vi "Application and database upload.vi"(8 "error in":errorcluster) -> (0 "error out":errorcluster, 1 ".dta file Path 2":path, 2 "Pass?":bool, 3 ".128 file Path 2":path)   [LabVIEW 2009]
uses:
  Digit IO PCI 6503/Digit IO control.ctl
  Global/Global 1.vi
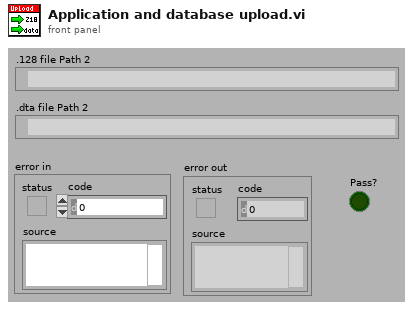
[diagram p1: front panel]
types:
  T1 = typedef "Digit IO control.ctl" = enum16{"Pull X1_4 Low", "Disconnect Pull X1_4 Low", "Down Cylinder", "Disconnect Down Cylinder", "Load X1_1_5", "Disconnect Load X1_1_5", "Measu X1_1_5", "Disconnect Measu X1_1_5", "Measu Z1_1_5", "Disconnect Measu Z1_1_5", "Power X1_1", "Disconnect Power X1_1", "RS232 Power", "Disconnect RS232 Power", "Card Cylinder", "Disconnect Card Cylinder", "Fail LED", "Disconnect Fail LED", "LCA Power", "Disconnect LCA Power", "BeyondCylinderDowndigit", "Disconnect BeyondCylinderDowendigit", "Frequency", "Disconnect Frequency", "Measu Current", "Disconnect Measu Current", "Measu current_1", "Disconnect Measu current_1", "Digit ALL", "Disconnect Digit ALL", "PASS LED", "Disconnect PASS LED", "Load Z1_1_3", "Disconnect Load Z1_1_3", "RS232 Connect", "Disconnect RS232 Connect", "Power Z1_7", "Disconnect Power Z1_7", "Pull Z_1_5  low", "Disconnect Pull Z_1_5  low", "Connect LCA_1", "Disconnect LCA_1", "short LCA", "Disconnect short LCA", "PT100", "Disconnect PT100", "NO connect", "Disconnect NO connect"}
  T2 = enum16{"Initialize", "Uploading 218 file", "Wait APPWAIT", "Uploading dta file", "Wait DBWATI", "Finish"}
  T3 = cluster{".128 file":path, "Appliction firmware file":path, "Data file":path, "Txt path":path, "EXCEL path":path}
  T4 = cluster{"VHEATFUSENOLOADMIN":string, "VHEATFUSELOADMAX":string, "VOVERRIDEDIODEMIN":string, "TDIFFMAX":string, "MEASFREQMAX":string, "MEASFREQMIN":string, "VOVER":string, "VMIDDLE":string, "VUNDER":string, "VNORESET":string, "VRESET":string, "WAITPING":string, "LRFID":string, "RFIDUID":string, "EXTEESIZE":string, "LCUTYPE":string, "LCUSUBTYPE":string, "TEVN":string, "BOOTVER":string, "APPVER":string, "ISLEEPMAX":string, "TSLEEP":string, "APPWAIT":string, "DBWAIT":string}
  T5 = cluster{"People":string, "product  number":string, "Test time":string, "VHeatFuse_noload":string, "VHeatFuse_load":string, "VoverrideDiode":string, "Test firmware upload via X1":string, "TemperAddress":string, "Troom":string, "TLCU":string, "Adjustment factor":string, "MeasuredFreq":string, "I2C communication":string, "Light-emitting diode on Z2":string, "Battery warning/inhibit":string, "Reset by IC10":string, "External EEPROM":string, "RFID card detection and reading RFID":string, "Production parameters in internal EEPROM":string, "Current consumption in sleep mode":string, "Application and database upload":string, "Test result":string, "Table head[22]":string, "Table head[23]":string}
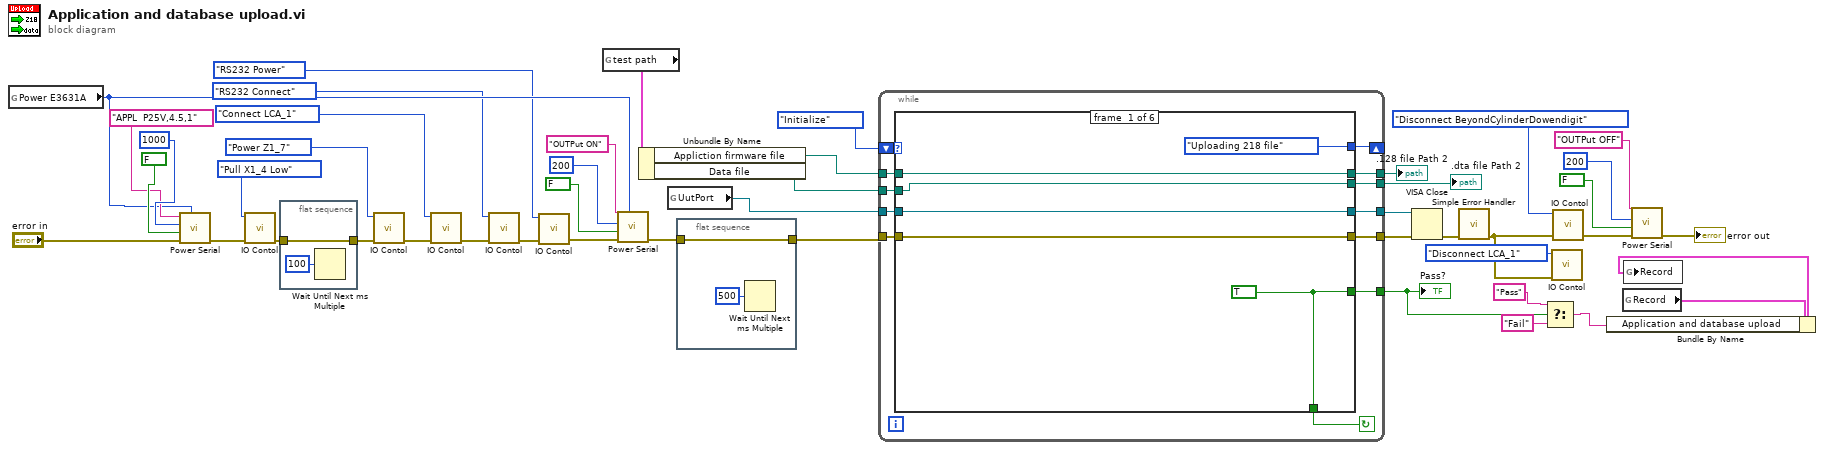
[diagram p0: block diagram]
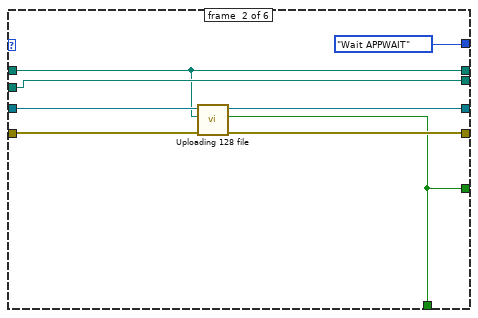
[diagram p2: hidden frame]
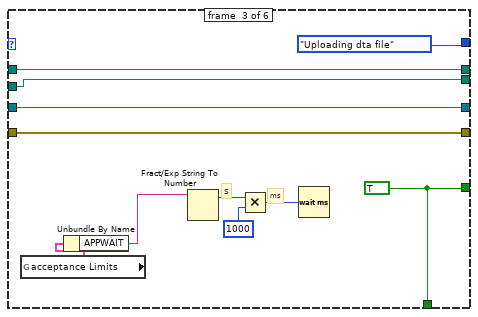
[diagram p3: hidden frame]
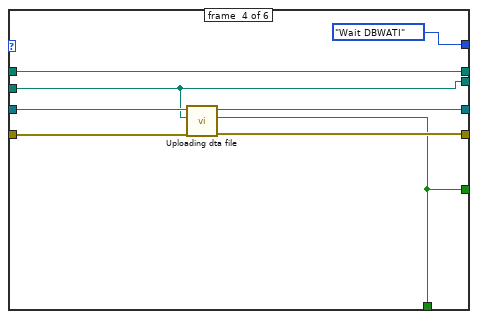
[diagram p4: hidden frame]
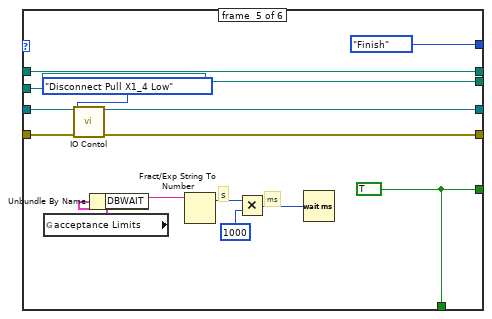
[diagram p5: hidden frame]
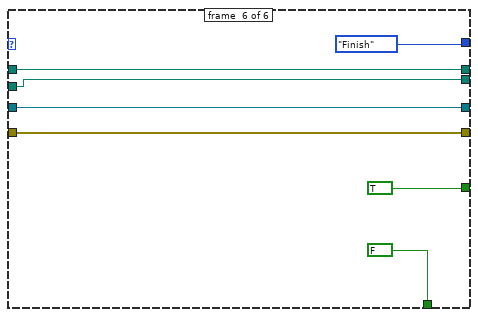
[diagram p6: hidden frame]
diagram:
  n1 = global read "Global 1.vi" "Power E3631A"() -> (w32:i32)
  n2 = call "Power Serial.vi"("VISA Resource Address"=w32, "error in (no error)"="error in", "Rd?"=FALSE, "Delay"=1000, "IN"="APPL  P25V,4.5,1" ("In")) -> ("error out"=w31:errorcluster)  [unwired: 6 out]
  n3 = call "IO Contol.vi"("error in"=w31, "IO Operation"=Digit_IO_control."Pull X1_4 Low" ("Enum")) -> ("error out"=w24:errorcluster)  [unwired: 9 out]
  n4 = flat-sequence {
    tunnel: w24 -> [w48]
    tunnel: [w48] -> w23
    frame #0 {
      n5 = Wait Until Next ms Multiple(millisecond multiple=u32 100) -> ()  [unwired: 1 out]
    }
  }
  n6 = call "IO Contol.vi"("error in"=w23, "IO Operation"=Digit_IO_control."Power Z1_7" ("Enum")) -> ("error out"=w1:errorcluster)  [unwired: 9 out]
  n7 = call "IO Contol.vi"("error in"=w1, "IO Operation"=Digit_IO_control."Connect LCA_1") -> ("error out"=w2:errorcluster)  [unwired: 9 out]
  n8 = call "IO Contol.vi"("error in"=w2, "IO Operation"=Digit_IO_control."RS232 Connect" ("Enum")) -> ("error out"=w30:errorcluster)  [unwired: 9 out]
  n9 = call "IO Contol.vi"("error in"=w30, "IO Operation"=Digit_IO_control."RS232 Power") -> ("error out"=w28:errorcluster)  [unwired: 9 out]
  n10 = global read "Global 1.vi" "test path"() -> (w7:T3)
  n11 = call "Power Serial.vi"("VISA Resource Address"=w32, "error in (no error)"=w28, "Rd?"=FALSE, "Delay"=200, "IN"="OUTPut ON" ("In")) -> ("error out"=w14:errorcluster)  [unwired: 6 out]
  n12 = Unbundle By Name(w7) -> ("Appliction firmware file"=w6:path, "Data file"=w5:path)
  n13 = global read "Global 1.vi" "UutPort"() -> (w12:refnum<visa-resource-name>)
  n14 = flat-sequence {
    tunnel: w14 -> [w50]
    tunnel: [w50] -> w13
    frame #0 {
      n15 = Wait Until Next ms Multiple(millisecond multiple=u32 500) -> ()  [unwired: 1 out]
    }
  }
  n16 = while {
    shift-right: [w53] -> _
    shift-left: T2."Initialize" -> [w62]
    tunnel: w12 -> [w60]
    tunnel: w13 -> [w59]
    tunnel: [w58] -> w44
    tunnel: [w57] -> w43
    tunnel: [w56] -> w20
    tunnel: w6 -> [w55]
    tunnel: w5 -> [w54]
    tunnel: [w52] -> w9
    tunnel: [w51] -> w8
    stop <- w61 continue-if-true
    n17 = case shown="\"Uploading dta file\"" w62 {
      tunnel: [T2."Uploading 218 file" T2."Wait APPWAIT" T2."Uploading dta file" T2."Wait DBWATI" T2."Finish" T2."Finish"] -> w53
      tunnel: [w66 w71 w87 w90 w107 FALSE] -> w61
      tunnel: w60 -> [w68 w75 w85 w94 w108 w115]
      tunnel: w59 -> [w67 w74 w84 w93 w102 w114]
      tunnel: [w68 w73 w85 w92 w108 w115] -> w58
      tunnel: [w67 w72 w84 w91 w98 w114] -> w57
      tunnel: [w66 w71 w87 w90 w107 TRUE] -> w56
      tunnel: w55 -> [w64 w69 w80 w88 w100 w110]
      tunnel: w54 -> [w63 w70 w79 w89 w99 w109]
      tunnel: [w64 w69 w80 w88 w100 w110] -> w52
      tunnel: [w63 w70 w79 w89 w99 w109] -> w51
      frame #0 {
        w66 = TRUE
      }
      frame #1 {
        n18 = call "Uploading 128 file.vi"("error in (no error)"=w74, ".128 file Path"=w69, "VISA resource name"=w75) -> ("error out"=w72:errorcluster, "Pass?"=w71:bool, "VISA resource name out"=w73:refnum<visa-resource-name>)  [unwired: 6 out]
      }
      frame #2 {
        w87 = TRUE
        # "s"
        # "ms"
        n19 = global read "Global 1.vi" "acceptance Limits"() -> (w78:T4)
        n20 = Unbundle By Name(w78) -> ("APPWAIT"=w77:string)
        n21 = Fract/Exp String To Number(string=w77) -> (offset past number=w83:i32)  [unwired: 4 out]
        n22 = Multiply(x=w83, y=1000) -> (x*y=w82:i32)
        n23 = Wait (ms)(milliseconds to wait=w82) -> ()  [unwired: 1 out]
      }
      frame #3 {
        n24 = call "Uploading dta file.vi"("error in (no error)"=w93, ".dta file Path"=w89, "VISA resource name"=w94) -> ("error out"=w91:errorcluster, "Pass?"=w90:bool, "VISA resource name out"=w92:refnum<visa-resource-name>)  [unwired: 6 out]
      }
      frame #4 {
        w107 = TRUE
        # "s"
        # "ms"
        n25 = global read "Global 1.vi" "acceptance Limits"() -> (w97:T4)
        n26 = call "IO Contol.vi"("error in"=w102, "IO Operation"=Digit_IO_control."Disconnect Pull X1_4 Low") -> ("error out"=w98:errorcluster)  [unwired: 9 out]
        n27 = Unbundle By Name(w97) -> ("DBWAIT"=w96:string)
        n28 = Fract/Exp String To Number(string=w96) -> (offset past number=w105:i32)  [unwired: 4 out]
        n29 = Multiply(x=w105, y=1000) -> (x*y=w103:i32)
        n30 = Wait (ms)(milliseconds to wait=w103) -> ()  [unwired: 1 out]
      }
      frame #5 {
      }
    }
  }
  "Pass?" <- w20
  ".128 file Path 2" <- w9
  ".dta file Path 2" <- w8
  n31 = VISA Close(VISA resource name=w44, error in (no error)=w43) -> (error out=w45:errorcluster)
  n32 = call <vilib>:"Simple Error Handler.vi"("error in (no error)"=w45) -> ("error out"=w11:errorcluster)  [unwired: 1 in, 7 out]
  n33 = Select(t="Pass", s=w20, f="Fail") -> (s? t:f=w15:string)
  n34 = call "IO Contol.vi"("error in"=w11, "IO Operation"=Digit_IO_control."Disconnect LCA_1") -> ()  [unwired: 10 out]
  n35 = call "IO Contol.vi"("error in"=w11, "IO Operation"=Digit_IO_control."Disconnect BeyondCylinderDowendigit") -> ("error out"=w39:errorcluster)  [unwired: 9 out]
  n36 = global read "Global 1.vi" "Record"() -> (w17:T5)
  n37 = Bundle By Name(cluster=w17, "Application and database upload"=w15) -> (w16:T5)
  n38 = global write "Global 1.vi" "Record"(w16) -> ()
  n39 = call "Power Serial.vi"("error in (no error)"=w39, "Rd?"=FALSE, "Delay"=200, "IN"="OUTPut OFF" ("In")) -> ("error out"=→"error out":errorcluster)  [unwired: 1 in, 6 out]
